vi "setUp.vi"(8 "error in (no error)":errorcluster, 11 "reference in":refnum<class "FPGA Register IO Tests.lvclass">) -> (0 "error out":errorcluster, 3 "reference out":refnum<class "FPGA Register IO Tests.lvclass">)   [LabVIEW 2020, in "FPGA Register IO Tests.lvclass"]
doc: "setUp runs prior to the test method during test execution. Use this method to initialize any object data required by your tests."
uses:
  FPGA Register IO Tests.lvclass
  C:/Program Files (x86)/National Instruments/LabVIEW 2020/vi.lib/addons/_JKI Toolkits/VI Tester/TestCase.llb/TestCase.lvclass
  FPGA Register IO Tests.lvclass/FPGA Register IO Tests.ctl
  <vilib>/addons/_JKI Toolkits/VI Tester/TestCase.llb/TestCase.lvclass
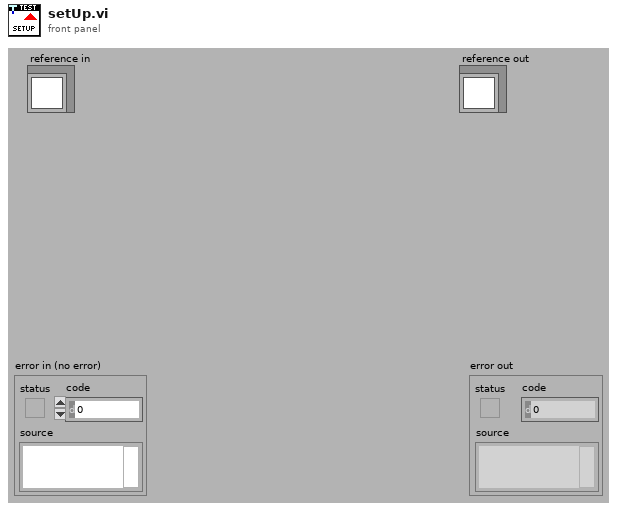
[diagram p1: front panel]
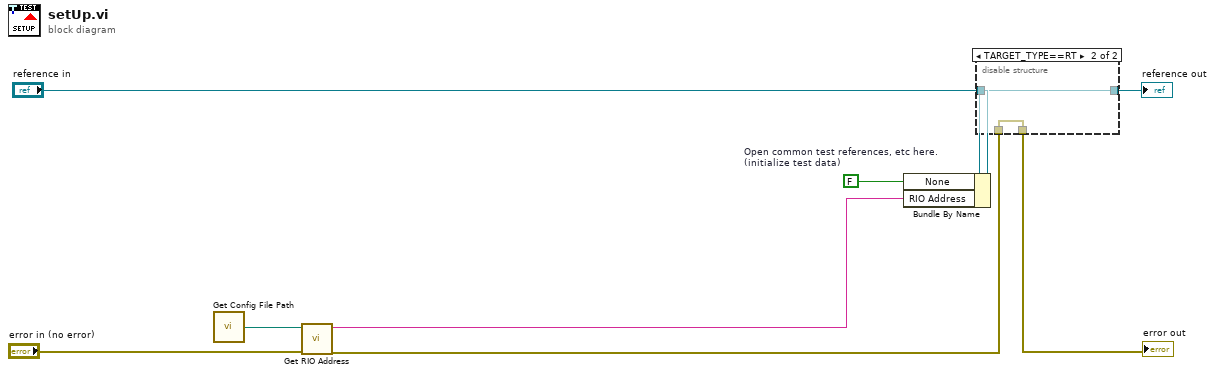
[diagram p0: block diagram]
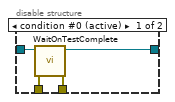
[diagram p2: hidden frame]
diagram:
  w5 = FALSE  # Open common test references, etc here. (initialize test data)
  n1 = call "Get Config File Path.vi"() -> ("config file path out"=w4:path)  [unwired: 1 in]
  n2 = call "Get RIO Address.vi"("error in (no error)"="error in (no error)", "configuration file path"=w4) -> ("error out"=w1:errorcluster, "RIO address out"=w2:string)  [unwired: 8 in]
  n3 = Bundle By Name(cluster="reference in", "None"=w5, "RIO Address"=w2) -> (w6:refnum<class "FPGA Register IO Tests.lvclass">)
  n4 = disable-structure shown="TARGET_TYPE==RT" {
    disable-tunnel: w1 -> [w13 w14]
    disable-tunnel: [w12 w14] -> w9
    disable-tunnel: [w11 w15] -> w7
    disable-tunnel: w6 -> [w10 w15]
    frame condition #0 (active) {
      n5 = call <vilib>:"WaitOnTestComplete.vi"("error in (no error)"=w13, "TestCase in"=w10) -> ("error out"=w12:errorcluster, "TestCase out"=w11:refnum<class "FPGA Register IO Tests.lvclass">)  [unwired: 8 in]
    }
    frame condition #1 {
    }
  }
  "error out" <- w9
  "reference out" <- w7
